vi "Read Hand_Type_Enum.vi"(8 "error in (no error)":errorcluster, 11 "CardHand in":refnum<class "CardHand.lvclass">) -> (0 "error out":errorcluster, 2 "Hand_Type_Enum":T1(ring), 3 "CardHand out":refnum<class "CardHand.lvclass">)   [LabVIEW 2021, in "2023.lvlib" / "CardHand.lvclass"]
uses:
  CardHand.lvclass
  CardHand.lvclass/CardHand.ctl
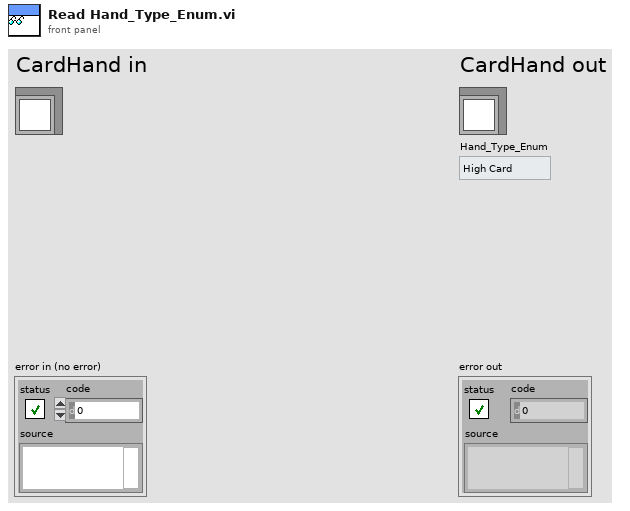
[diagram p1: front panel]
types:
  T1 = enum16{"High Card", "One Pair", "Two Pair", "Three of Kind", "Full House", "Four of Kind", "Five of Kind", "ERROR"}
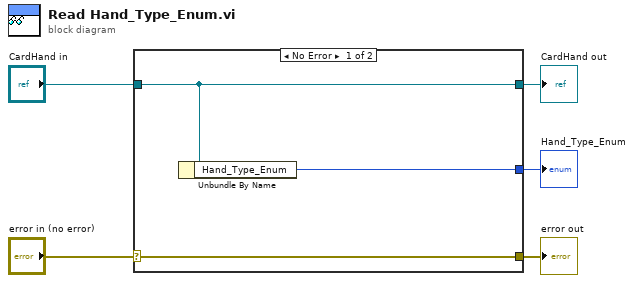
[diagram p0: block diagram]
diagram:
  n1 = case shown="No Error" "error in (no error)" {
    selector: "error in (no error)" -> [w8 w9]
    tunnel: [w8 w9] -> w4
    tunnel: [w7 w10] -> w2
    tunnel: "CardHand in" -> [w7 w10]
    tunnel: [w6 _] -> w1
    frame No Error {
      n2 = Unbundle By Name(w7) -> ("Hand_Type_Enum"=w6:T1)
    }
    frame Error {
    }
  }
  "error out" <- w4
  "CardHand out" <- w2
  "Hand_Type_Enum" <- w1
